vi "SetupTiming.vi"(8 "error in (no error)":errorcluster, 11 "ClassIn":refnum<class "NiPxi6123.lvclass">) -> (0 "error out":errorcluster, 3 "ClassOut":refnum<class "NiPxi6123.lvclass">)   [LabVIEW 2014, in "SamplerPlugins.lvlib" / "NiPxi6123.lvclass"]
uses:
  NiPxi6123.lvclass
  NiPxi6123.lvclass/NiPxi6123.ctl
  Accessors/Read sample mode.vi
  <vilib>/Utility/error.llb/Error Cluster From Error Code.vi
  <vilib>/DAQmx/configure/timing.llb/DAQmx Timing (Sample Clock).vi
  <vilib>/ErrorRing/Error Ring.xnode
  <resource>/objmgr/daqmx.rc
panel:
  out "sample mode":i32(ring)=10178 items=["Finite Samples"=10178, "Continuous Samples"=10123, "Hardware Timed Single Point"=12522]
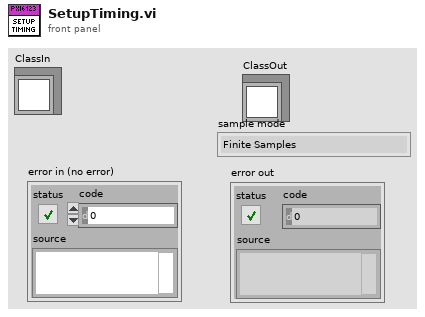
[diagram p1: front panel]
types:
  T1 = typedef "SamplerPlugins.lvlib/SamplerPluginsBase.lvclass/ConfigMultiPointParams.ctl" = cluster{"iTriggerCount":i32, "iSampleCount":i32, "eSampleClock":u16, "dSampleInterval":dbl}
  T2 = typedef "SamplerPlugins.lvlib/SamplerPluginsBase.lvclass/TriggerParams.ctl" = cluster{"eEdge":u16, "sSource":string}
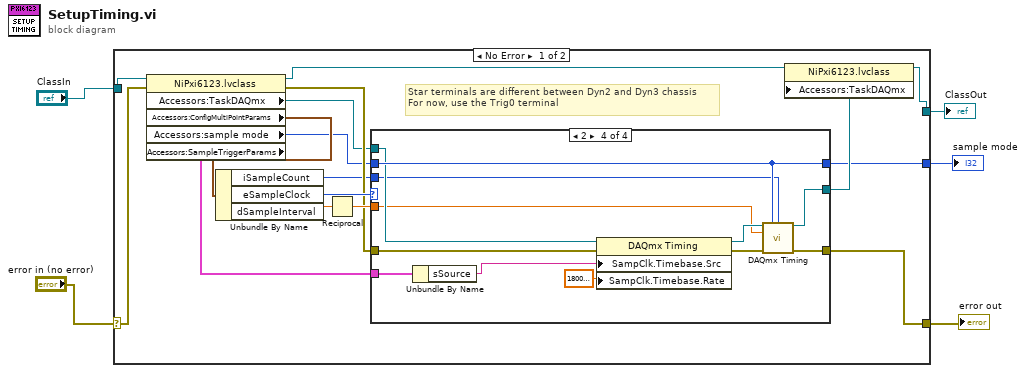
[diagram p0: block diagram]
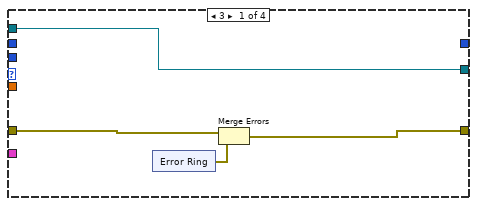
[diagram p2: hidden frame]
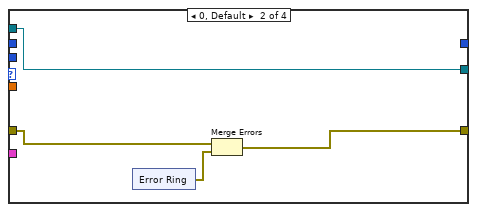
[diagram p3: hidden frame]
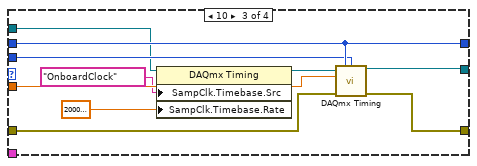
[diagram p4: hidden frame]
diagram:
  n1 = case shown="No Error" "error in (no error)" {
    selector: "error in (no error)" -> [w10 w62]
    tunnel: [w21 w63] -> w4
    tunnel: "ClassIn" -> [w11 w63]
    tunnel: [w17 w62] -> w2
    tunnel: [w9 _] -> w1
    frame No Error {
      # "Star terminals are different between Dyn2 and Dyn3 chassis\nFor now, use the Trig0 terminal"
      n2 = property class="NiPxi6123.lvclass"(reference=w11, error in=w10) -> (reference out=w16:refnum<class "NiPxi6123.lvclass">, error out=w15:errorcluster, "Accessors:TaskDAQmx"=w14:refnum<k21>, "Accessors:ConfigMultiPointParams"=w13:T1, "Accessors:sample mode"=w12:i32, "Accessors:SampleTriggerParams"=w6:T2)
      n3 = Unbundle By Name(w13) -> ("iSampleCount"=w8:i32, "eSampleClock"=w20:u16, "dSampleInterval"=w7:dbl)
      n4 = Reciprocal(x=w7) -> (1/x=w19:dbl)
      n5 = case shown="2" w20 {
        tunnel: w15 -> [w25 w34 w44 w54]
        tunnel: w12 -> [_ _ w49 w60]
        tunnel: w14 -> [w23 w31 w41 w59]
        tunnel: w19 -> [_ _ w48 w52]
        tunnel: w8 -> [_ _ w47 w57]
        tunnel: [w23 w31 w46 w56] -> w18
        tunnel: [w24 w33 w45 w55] -> w17
        tunnel: [_ _ w49 w60] -> w9
        tunnel: w6 -> [_ _ _ w51]
        frame 3 {
          n6 = xnode "Error Ring"() -> ("error out"=w22:errorcluster)
          n7 = Merge Errors(w25, w22) -> (w24:errorcluster)
        }
        frame 0, Default {
          n8 = xnode "Error Ring"() -> ("error out"=w32:errorcluster)
          n9 = Merge Errors(w34, w32) -> (w33:errorcluster)
        }
        frame 10 {
          n10 = property class="DAQmx Timing"(reference=w41, "SampClk.Timebase.Src"=tag "OnboardClock" ("source"), "SampClk.Timebase.Rate"=20000000.0 ("f")) -> (reference out=w40:refnum<k21>)  [unwired: 1 in, 1 out]
          n11 = call-poly <vilib>:"DAQmx Timing.vi"("task/channels in"=w40, "sample mode"=w49, "samples per channel"=w47, "rate"=w48, "error in"=w44) -> ("task out"=w46:refnum<k21>, "error out"=w45:errorcluster)  [unwired: 9 in]
        }
        frame 2 {
          n12 = Unbundle By Name(w51) -> ("sSource"=w50:string)
          n13 = property class="DAQmx Timing"(reference=w59, error in=w54, "SampClk.Timebase.Src"=w50, "SampClk.Timebase.Rate"=18000000.0 ("f")) -> (reference out=w61:refnum<k21>, error out=w58:errorcluster)
          n14 = call-poly <vilib>:"DAQmx Timing.vi"("task/channels in"=w61, "sample mode"=w60, "samples per channel"=w57, "rate"=w52, "error in"=w58) -> ("task out"=w56:refnum<k21>, "error out"=w55:errorcluster)  [unwired: 9 in]
        }
      }
      n15 = property class="NiPxi6123.lvclass"(reference=w16, "Accessors:TaskDAQmx"=w18) -> (reference out=w21:refnum<class "NiPxi6123.lvclass">)  [unwired: 1 in, 1 out]
    }
    frame Error {
    }
  }
  "ClassOut" <- w4
  "error out" <- w2
  "sample mode" <- w1
